vi "d1000 start t move.vi"(6 "Tacc":dbl, 7 "MaxVel":i32, 9 "StrVel":i32, 10 "Dist":i32, 11 "axis":i16) -> (3 "function return":u32)   [LabVIEW 2019, in "Dmc1000.lvlib"]
doc: "DMC1000_API DWORD WINAPI d1000_start_t_move(short axis,long Dist, long StrVel,long MaxVel,double Tacc);"
uses:
  Dmc1000.lvlib
  Dmc1000.dll
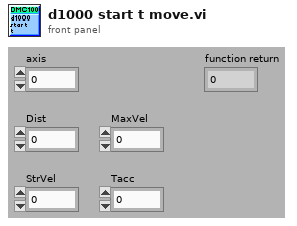
[diagram p1: front panel]
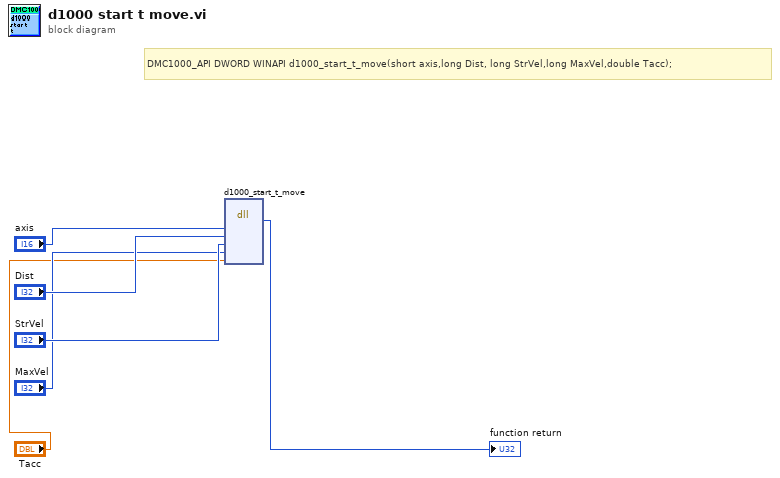
[diagram p0: block diagram]
diagram:
  # "DMC1000_API DWORD WINAPI d1000_start_t_move(short axis,long Dist, long StrVel,long MaxVel,double Tacc);"
  n1 = dll-call lib="C:/Users/Admin/Desktop/Standar Program/System/LLB/DMC1000B/Dmc1000.*" fn="d1000_start_t_move"("axis"="axis", "Dist"="Dist", "StrVel"="StrVel", "MaxVel"="MaxVel", "Tacc"="Tacc") -> (→"function return":u32)  [unwired: 8 in, 2 out]
